vi "main.playground.vi"() -> ()   [LabVIEW 2016]
uses:
  KeyenceCVX.CodeDetails.ctl
  KeyenceCVX.Data.Status.ctl
  KeyenceCVX.Data.Status.State.ctl
  private/controls/TriggerNo.ctl
  private/controls/RunMode.ctl
  KeyenceCVX.ChangeProgram.Data.ctl
  Keyence/LowLevel/Keyence.Global.vi
panel:
  in  "TriggerNo":T1=1 items=["1"=1, "2"=2, "3"=3, "4"=4, "ALL"=5]
  in  "Boolean":bool=TRUE
  out "CVX Status":T2 {"TriggerNo" items=["1"=1, "2"=2, "3"=3, "4"=4, "ALL"=5]}
  out "CVX Readout details":T5
  in  "Reboot?":bool=TRUE
  in  "ProgramNumber":u16
  in  "RESET":bool
  in  "stop":bool
  in  "Trigger":bool
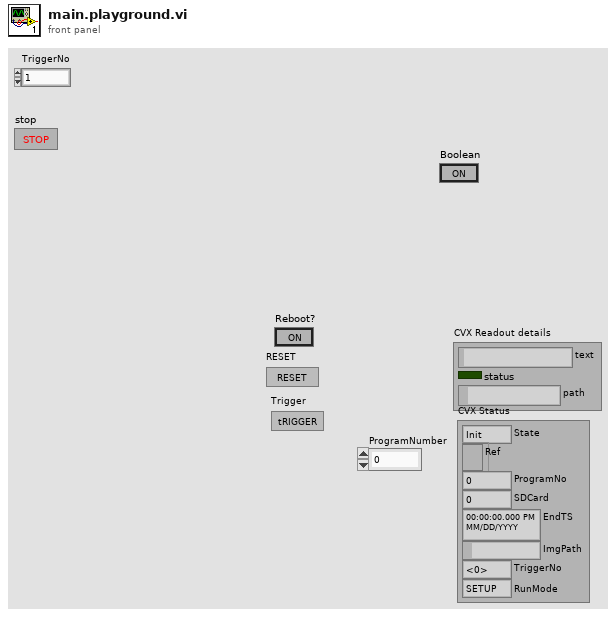
[diagram p1: front panel]
types:
  T1 = typedef "TriggerNo.ctl" = u8
  T2 = typedef "KeyenceCVX.Data.Status.ctl" = cluster{"State":T3, "Ref":refnum<k5>, "ProgramNo":u16, "SDCard":u8, "EndTS":timestamp, "ImgPath":path, "TriggerNo":T1, "RunMode":T4}
  T3 = typedef "KeyenceCVX.Data.Status.State.ctl" = enum16{"Init", "Idle", "Scan", "Reset", "ScanAck", "ChangeProgram"}
  T4 = typedef "RunMode.ctl" = enum16{"SETUP", "RUN"}
  T5 = typedef "KeyenceCVX.CodeDetails.ctl" = cluster{"text":string, "status":bool, "path":path}
  T6 = typedef "KeyenceCVX.ChangeProgram.Data.ctl" = cluster{"SDCard":u8, "ProgramNo":u16}
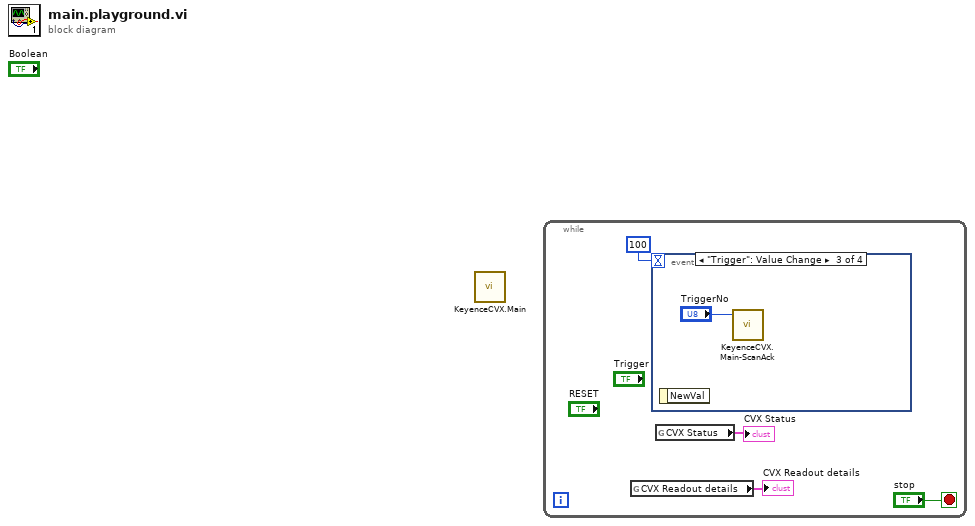
[diagram p0: block diagram]
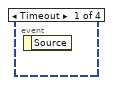
[diagram p2: hidden frame]
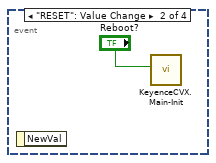
[diagram p3: hidden frame]
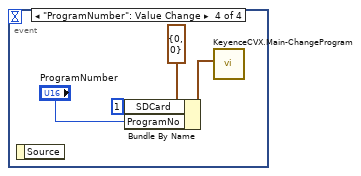
[diagram p4: hidden frame]
diagram:
  n1 = call "KeyenceCVX.Main.vi"() -> ()  [unwired: 12 in]
  n2 = while {
    stop <- "stop" stop-if-true
    n3 = global read "Keyence.Global.vi" "CVX Readout details"() -> (→"CVX Readout details":T5)
    n4 = event shown="[2] \"Trigger\": Value Change" {
      selector: _ -> [_ _ _ _]
      dyn-events: _ -> [_ _ _ _]
      timeout: 100 -> [_ _ _ _]
      event Timeout {
        n5 = event-data() -> ()  [unwired: 1 in, 1 out]
      }
      event "RESET": Value Change {
        n6 = event-data() -> ()  [unwired: 1 in, 1 out]
        n7 = call "KeyenceCVX.Main-Init.vi"("restart (T)"="Reboot?") -> ()  [unwired: 10 in, 1 out]
      }
      event "Trigger": Value Change {
        n8 = event-data() -> ()  [unwired: 1 in, 1 out]
        n9 = call "KeyenceCVX.Main-ScanAck.vi"("TriggerNo"="TriggerNo") -> ()  [unwired: 8 in, 3 out]
      }
      event "ProgramNumber": Value Change {
        n10 = event-data() -> ()  [unwired: 1 in, 1 out]
        n11 = Bundle By Name(cluster=T6 {"SDCard"=0, "ProgramNo"=0} ("ChangeProgram.Data"), "SDCard"=u8 1, "ProgramNo"="ProgramNumber") -> (w7:T6)
        n12 = call "KeyenceCVX.Main-ChangeProgram.vi"("ChangeProgram.Data"=w7) -> ()  [unwired: 10 in, 1 out]
      }
    }
    n13 = global read "Keyence.Global.vi" "CVX Status"() -> (→"CVX Status":T2)
  }
